vi "关键参数交互.vi"(9 "量程选择":enum16{"低量程", "高量程"}(ring), 11 "模型":enum32{"线性", "多项式", "折线"}(ring)) -> ()   [LabVIEW 2016, in "斯坦道CODMn.lvlib"]
panel:
  out "x != y?":T1
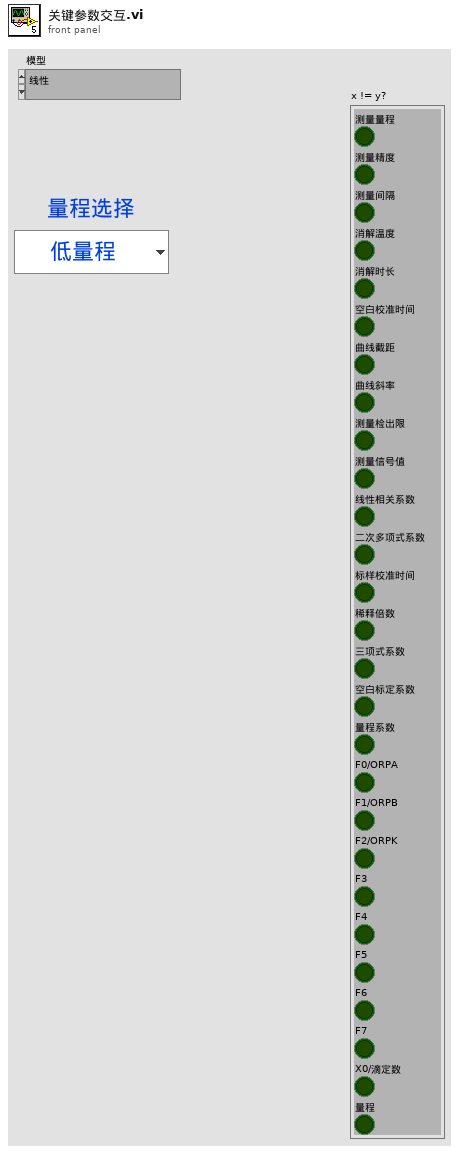
[diagram p1: front panel]
types:
  T1 = cluster{"测量量程":bool, "测量精度":bool, "测量间隔":bool, "消解温度":bool, "消解时长":bool, "空白校准时间":bool, "曲线截距":bool, "曲线斜率":bool, "测量检出限":bool, "测量信号值":bool, "线性相关系数":bool, "二次多项式系数":bool, "标样校准时间":bool, "稀释倍数":bool, "三项式系数":bool, "空白标定系数":bool, "量程系数":bool, "F0/ORPA":bool, "F1/ORPB":bool, "F2/ORPK":bool, "F3":bool, "F4":bool, "F5":bool, "F6":bool, "F7":bool, "X0/滴定数":bool, "量程":bool}
  T2 = cluster{"chose":string, "公式":cluster{"X^2":dbl, "X":dbl, "b":dbl}}
  T3 = cluster{"测量量程":dbl, "测量精度":dbl, "测量间隔":dbl, "消解温度":dbl, "消解时长":dbl, "空白校准时间":timestamp, "曲线截距":dbl, "曲线斜率":dbl, "测量检出限":dbl, "测量信号值":dbl, "线性相关系数":dbl, "二次多项式系数":dbl, "标样校准时间":timestamp, "稀释倍数":dbl, "三项式系数":dbl, "空白标定系数":dbl, "量程系数":dbl, "F0/ORPA":dbl, "F1/ORPB":dbl, "F2/ORPK":dbl, "F3":dbl, "F4":dbl, "F5":dbl, "F6":dbl, "F7":dbl, "X0/滴定数":dbl, "量程":dbl}
  T4 = cluster{"时间标识":timestamp, "设备":string, "日志信息":string, "流程参数":string}
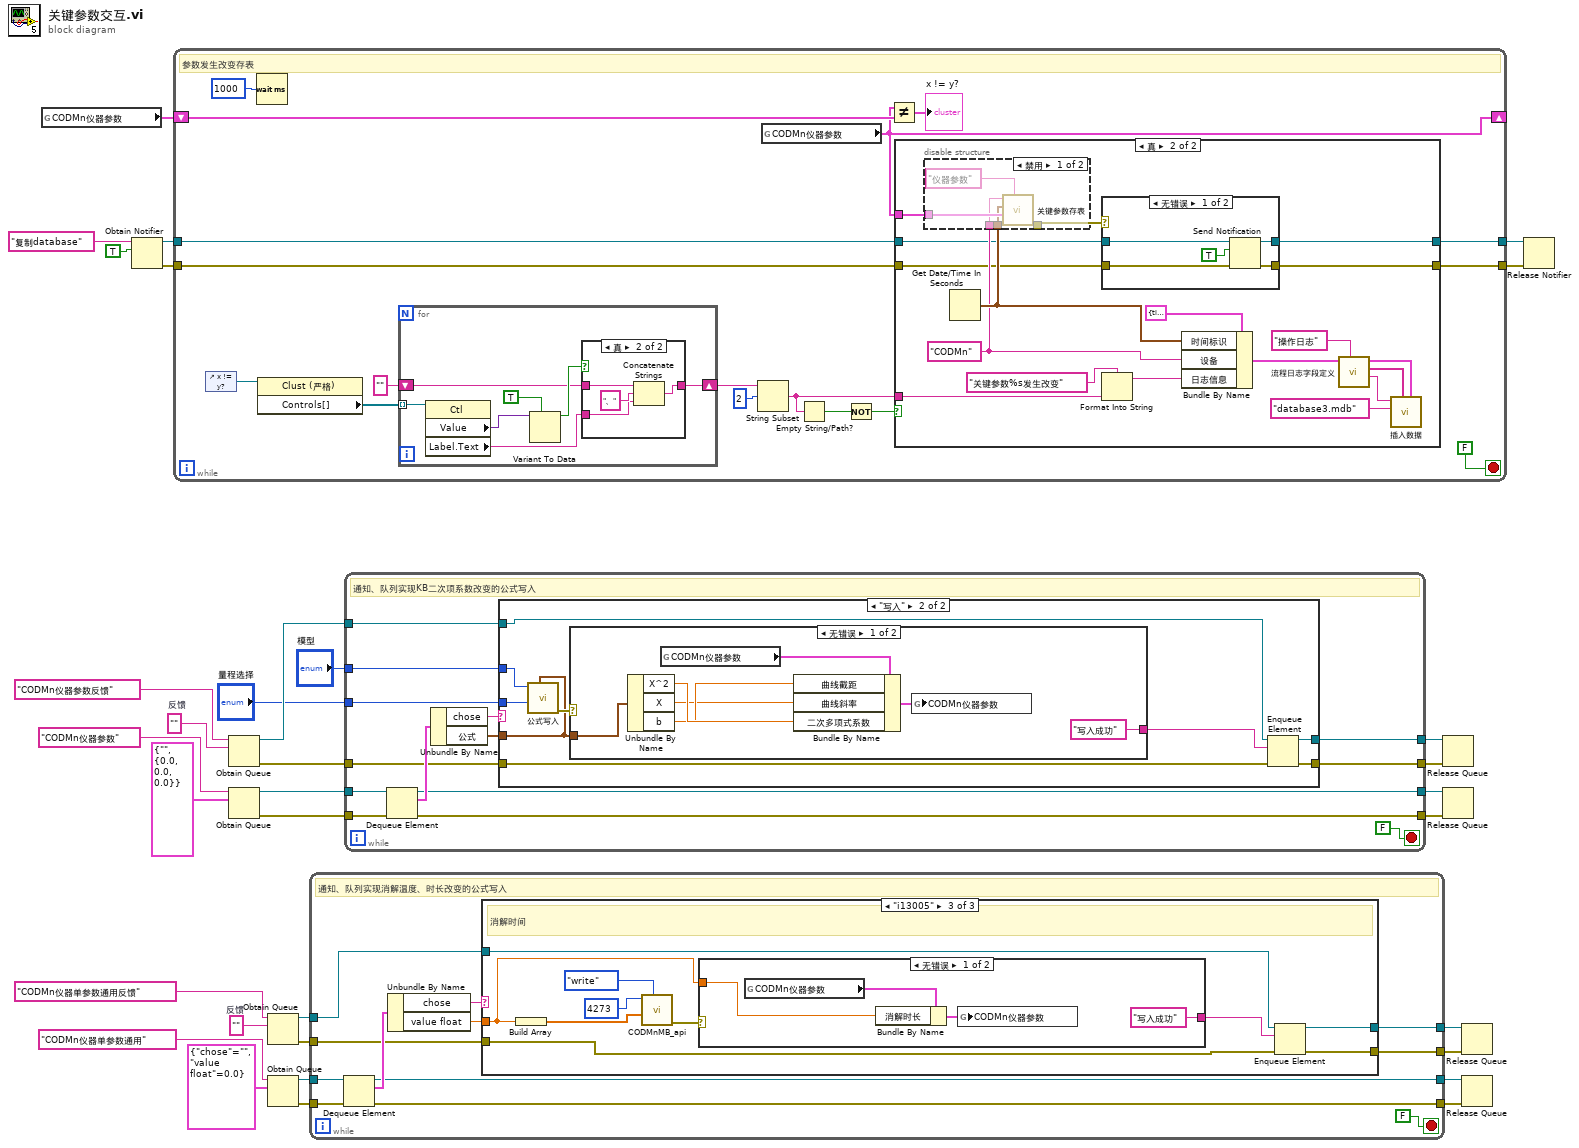
[diagram p0: block diagram]
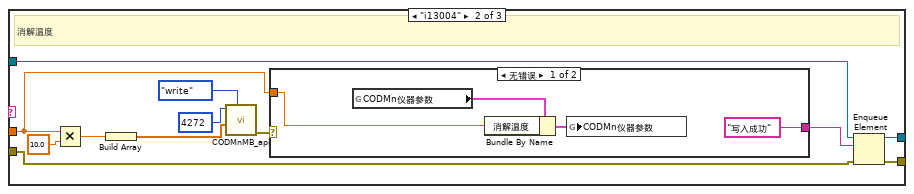
[diagram p3: hidden frame]
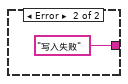
[diagram p4: hidden frame]
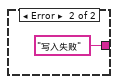
[diagram p5: hidden frame]
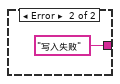
[diagram p7: hidden frame]
diagram:
  w9 = ""  # 反馈
  w24 = ""  # 反馈
  n1 = global read "CODMn断电保存全局变量.vi" "CODMn仪器参数"() -> (w33:T3)
  n2 = Obtain Notifier(name (unnamed)="复制database" ("名称（未命名）"), notification data type=TRUE) -> (notifier out=w18:refnum<notifier>, error out=w17:errorcluster)  [unwired: 2 in, 1 out]
  n3 = while {
    shift-right: [w45] -> _
    shift-left: w33 -> [w48]
    tunnel: w18 -> [w41]
    tunnel: w17 -> [w44]
    tunnel: [w43] -> w16
    tunnel: [w42] -> w15
    stop <- FALSE stop-if-true
    # "参数发生改变存表"
    n4 = control-ref of="x != y?"() -> (w46:refnum<vi>)
    n5 = Wait (ms)(milliseconds to wait=u32 1000 ("等待时间（毫秒）")) -> ()  [unwired: 1 out]
    n6 = property class="Clust (严格)"(reference=w46) -> ("Controls[]"=w36:refnum<vi>[])  [unwired: 1 in, 2 out]
    n7 = for {
      tunnel: w36 -> [w57] mode=indexing
      shift-right: [w51] -> w38
      shift-left: "" -> [w53]
      n8 = property class="Ctl"(reference=w57) -> ("Value"=w55:variant, "Label.Text"=w52:string)  [unwired: 1 in, 2 out]
      n9 = Variant To Data(type=TRUE, Variant=w55) -> (data=w54:bool)  [unwired: 1 in, 1 out]
      n10 = case shown="真" w54 {
        tunnel: w53 -> [w58 w62]
        tunnel: w52 -> [_ w59]
        tunnel: [w58 w61] -> w51
        frame False {
        }
        frame True {
          n11 = Concatenate Strings(w62, "、", w59) -> (w61:string)
        }
      }
    }
    n12 = String Subset(string=w38, offset (0)=2 ("偏移量(0)")) -> (substring=w34:string)  [unwired: 1 in]
    n13 = global read "CODMn断电保存全局变量.vi" "CODMn仪器参数"() -> (w45:T3)
    n14 = Empty String/Path?(string/path=w34) -> (empty?=w40:bool)
    n15 = Not(x=w40) -> (.not. x?=w35:bool)
    n16 = Not Equal?(x=w45, y=w48) -> (x != y?=→"x != y?":T1)
    n17 = case shown="真" w35 {
      tunnel: w45 -> [_ w82]
      tunnel: w34 -> [_ w77]
      tunnel: w44 -> [w64 w68]
      tunnel: [w63 w67] -> w43
      tunnel: [w64 w66] -> w42
      tunnel: w41 -> [w63 w65]
      frame False {
      }
      frame True {
        w79 = "CODMn" ("仪器名称")
        n18 = Get Date/Time In Seconds() -> (seconds since 1Jan1904=w80:timestamp)
        n19 = disable-structure shown="禁用" {
          disable-tunnel: w82 -> [w86 _]
          disable-tunnel: w80 -> [w85 _]
          disable-tunnel: w79 -> [w84 _]
          disable-tunnel: [w83 _] -> w69
          frame Disabled {
            n20 = call "关键参数存表.vi"("table"="仪器参数", "仪器参数"=w86, "datatime"=w85, "仪器名称"=w84) -> ("error out"=w83:errorcluster)  [unwired: 7 in]
          }
          frame Enabled {
          }
        }
        n21 = case shown="无错误" w69 {
          tunnel: w65 -> [w92 w94]
          tunnel: w68 -> [w91 w93]
          tunnel: [w89 w94] -> w67
          tunnel: [w88 w93] -> w66
          frame No Error {
            n22 = Send Notification(notification=TRUE ("通知"), notifier=w92, error in (no error)=w91) -> (notifier out=w89:refnum<notifier>, error out=w88:errorcluster)
          }
          frame Error {
          }
        }
        n23 = Format Into String(format string="关键参数%s发生改变" ("格式字符串"), w77) -> (resulting string=w76:string)  [unwired: 2 in, 1 out]
        n24 = Bundle By Name(cluster=T4 {"时间标识"=timestamp(0 s since 1904-01-01), "设备"="", "日志信息"="", "流程参数"=""} ("data in"), "时间标识"=w80, "设备"=w79, "日志信息"=w76) -> (w70:T4)
        n25 = call "流程日志字段定义.vi"("table输入"="操作日志", "data in"=w70) -> ("table输出"=w73:string, "columns"=w74:string[], "data out"=w75:T4)  [unwired: 7 in]
        n26 = call "插入数据.vi"("data"=w75, "columns"=w74, "database"="database3.mdb", "table"=w73) -> ()  [unwired: 7 in, 1 out]
      }
    }
  }
  n27 = Obtain Queue(name (unnamed)="CODMn仪器参数反馈" ("名称（未命名）"), element data type=w24) -> (queue out=w25:refnum<queue>, error out=w23:errorcluster)  [unwired: 3 in, 1 out]
  n28 = Obtain Queue(name (unnamed)="CODMn仪器参数" ("名称（未命名）"), element data type=T2 {"chose"="", "公式"={"X^2"=0.0, "X"=0.0, "b"=0.0}}) -> (queue out=w32:refnum<queue>, error out=w31:errorcluster)  [unwired: 3 in, 1 out]
  n29 = Obtain Queue(name (unnamed)="CODMn仪器单参数通用反馈" ("名称（未命名）"), element data type=w9) -> (queue out=w8:refnum<queue>, error out=w10:errorcluster)  [unwired: 3 in, 1 out]
  n30 = Obtain Queue(name (unnamed)="CODMn仪器单参数通用" ("名称（未命名）"), element data type=cluster{"chose":string, "value float":dbl} {"chose"="", "value float"=0.0}) -> (queue out=w1:refnum<queue>, error out=w2:errorcluster)  [unwired: 3 in, 1 out]
  n31 = while {
    tunnel: w1 -> [w105]
    tunnel: w2 -> [w104]
    tunnel: [w100] -> w5
    tunnel: [w99] -> w6
    tunnel: w8 -> [w98]
    tunnel: w10 -> [w97]
    tunnel: [w96] -> w11
    tunnel: [w95] -> w12
    stop <- FALSE stop-if-true
    # "通知、队列实现消解温度、时长改变的公式写入"
    n32 = Dequeue Element(queue=w105, error in (no error)=w104) -> (queue out=w100:refnum<queue>, element=w103:cluster{"chose":string, "value float":dbl}, error out=w99:errorcluster)  [unwired: 1 in, 1 out]
    n33 = Unbundle By Name(w103) -> ("chose"=w102:string, "value float"=w101:dbl)
    n34 = case shown="\"i13005\"" w102 {
      tunnel: w101 -> [_ w109 w126]
      tunnel: w98 -> [w108 w120 w135]
      tunnel: w97 -> [w107 w118 w131]
      tunnel: [w108 w117 w133] -> w96
      tunnel: [w107 w116 w132] -> w95
      frame "假", Default {
      }
      frame "i13004" {
        # "消解温度"
        n35 = Multiply(x=w109, y=10.0) -> (x*y=w112:dbl)
        n36 = Build Array(w112) -> (w111:dbl[])
        n37 = call "CODMnMB_api.vi"("STEP"=enum16{"open", "read", "write", "close"}."write", "values"=w111, "starting address"=u16 4272) -> ("error out"=w110:errorcluster)  [unwired: 6 in, 2 out]
        n38 = case shown="无错误" w110 {
          tunnel: ["写入成功" ("消息") "写入失败" ("消息")] -> w119
          tunnel: w109 -> [w121 _]
          frame No Error {
            n39 = global read "CODMn断电保存全局变量.vi" "CODMn仪器参数"() -> (w123:T3)
            n40 = Bundle By Name(cluster=w123, "消解温度"=w121) -> (w122:T3)
            n41 = global write "CODMn断电保存全局变量.vi" "CODMn仪器参数"(w122) -> ()
          }
          frame Error {
          }
        }
        n42 = Enqueue Element(queue=w120, element=w119, error in (no error)=w118) -> (queue out=w117:refnum<queue>, error out=w116:errorcluster)  [unwired: 1 in, 1 out]
      }
      frame "i13005" {
        # "消解时间"
        n43 = Build Array(w126) -> (w128:dbl[])
        n44 = call "CODMnMB_api.vi"("STEP"=enum16{"open", "read", "write", "close"}."write", "values"=w128, "starting address"=u16 4273) -> ("error out"=w127:errorcluster)  [unwired: 6 in, 2 out]
        n45 = case shown="无错误" w127 {
          tunnel: ["写入成功" ("消息") "写入失败" ("消息")] -> w134
          tunnel: w126 -> [w137 _]
          frame No Error {
            n46 = global read "CODMn断电保存全局变量.vi" "CODMn仪器参数"() -> (w138:T3)
            n47 = Bundle By Name(cluster=w138, "消解时长"=w137) -> (w136:T3)
            n48 = global write "CODMn断电保存全局变量.vi" "CODMn仪器参数"(w136) -> ()
          }
          frame Error {
          }
        }
        n49 = Enqueue Element(queue=w135, element=w134, error in (no error)=w131) -> (queue out=w133:refnum<queue>, error out=w132:errorcluster)  [unwired: 1 in, 1 out]
      }
    }
  }
  n50 = while {
    tunnel: w32 -> [w153]
    tunnel: w31 -> [w152]
    tunnel: [w148] -> w28
    tunnel: [w147] -> w27
    tunnel: w25 -> [w146]
    tunnel: w23 -> [w145]
    tunnel: [w144] -> w22
    tunnel: [w143] -> w21
    tunnel: "模型" -> [w142]
    tunnel: "量程选择" -> [w141]
    stop <- FALSE stop-if-true
    # "通知、队列实现KB二次项系数改变的公式写入"
    n51 = Dequeue Element(queue=w153, error in (no error)=w152) -> (queue out=w148:refnum<queue>, element=w151:T2, error out=w147:errorcluster)  [unwired: 1 in, 1 out]
    n52 = Unbundle By Name(w151) -> ("chose"=w150:string, "公式"=w149:cluster{"X^2":dbl, "X":dbl, "b":dbl})
    n53 = case shown="\"写入\"" w150 {
      tunnel: w149 -> [_ w158]
      tunnel: w146 -> [w156 w165]
      tunnel: w145 -> [w155 w163]
      tunnel: [w156 w162] -> w144
      tunnel: [w155 w161] -> w143
      tunnel: w142 -> [_ w159]
      tunnel: w141 -> [_ w157]
      frame "假", Default {
      }
      frame "写入" {
        n54 = call "公式写入.vi"("公式"=w158, "量程选择"=w157, "模型"=w159) -> ("error out"=w160:errorcluster)  [unwired: 8 in]
        n55 = case shown="无错误" w160 {
          tunnel: ["写入成功" ("消息") "写入失败" ("消息")] -> w164
          tunnel: w158 -> [w166 _]
          frame No Error {
            n56 = Unbundle By Name(w166) -> ("X^2"=w169:dbl, "X"=w167:dbl, "b"=w168:dbl)
            n57 = global read "CODMn断电保存全局变量.vi" "CODMn仪器参数"() -> (w170:T3)
            n58 = Bundle By Name(cluster=w170, "曲线截距"=w168, "曲线斜率"=w167, "二次多项式系数"=w169) -> (w171:T3)
            n59 = global write "CODMn断电保存全局变量.vi" "CODMn仪器参数"(w171) -> ()
          }
          frame Error {
          }
        }
        n60 = Enqueue Element(queue=w165, element=w164, error in (no error)=w163) -> (queue out=w162:refnum<queue>, error out=w161:errorcluster)  [unwired: 1 in, 1 out]
      }
    }
  }
  n61 = Release Queue(queue=w22, error in (no error)=w21) -> ()  [unwired: 1 in, 3 out]
  n62 = Release Queue(queue=w28, error in (no error)=w27) -> ()  [unwired: 1 in, 3 out]
  n63 = Release Queue(queue=w11, error in (no error)=w12) -> ()  [unwired: 1 in, 3 out]
  n64 = Release Queue(queue=w5, error in (no error)=w6) -> ()  [unwired: 1 in, 3 out]
  n65 = Release Notifier(notifier=w16, error in (no error)=w15) -> ()  [unwired: 1 in, 3 out]
